vi "Template Replace.vi"() -> ()   [LabVIEW 2013]
panel:
  in  "String 6":string="fasdfas"
  out "Boolean 5":bool=TRUE
  in  "Boolean 4":bool
  out "Boolean 3":bool
  out "Numeric 2":dbl
  in  "Numeric":u16 format="%.0x"
  out "Cluster":cluster{"Boolean 2":bool}
  out "Array":string[](array[string])
  in  "Error In":errorcluster
  in  "String 5":string
  out "String 4":string
  in  "File Path Control":path
  in  "String 3":string="324"
  out "String 2":string
  in  "String":string
  out "Boolean 2":bool
  in  "Boolean":bool
  in  "Cluster 3":T1
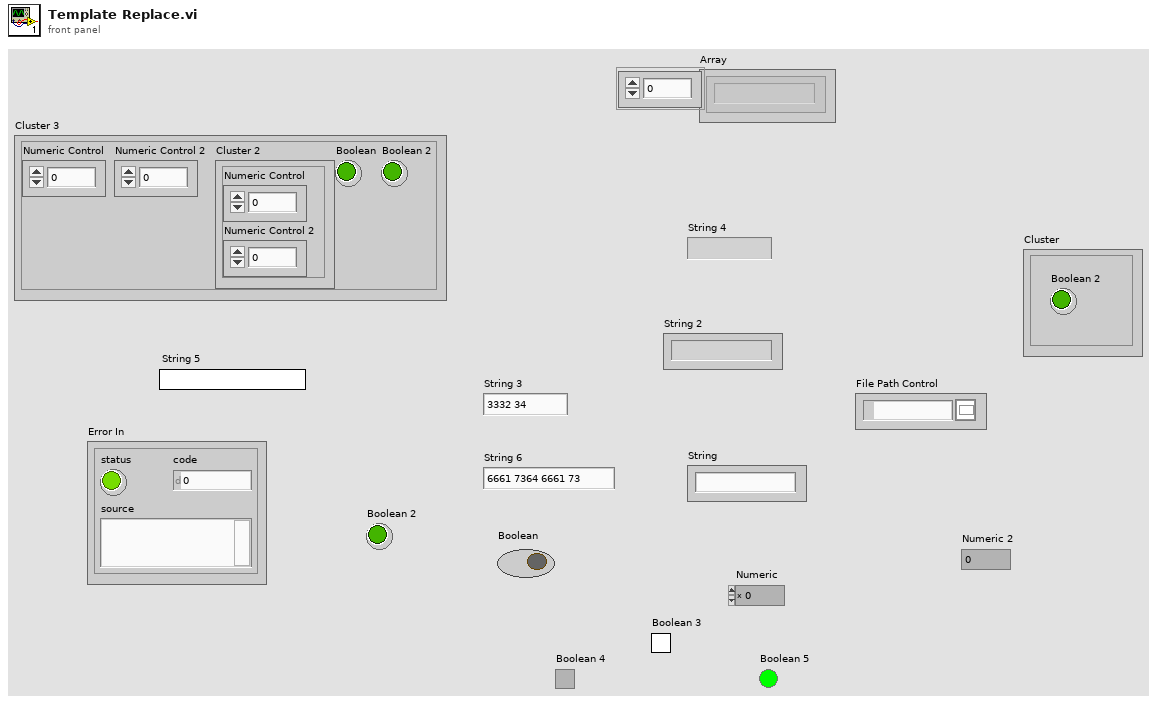
[diagram p1: front panel]
types:
  T1 = cluster{"Numeric Control":dbl, "Numeric Control 2":dbl, "Cluster 2":cluster{"Numeric Control":dbl, "Numeric Control 2":dbl}, "Boolean":bool, "Boolean 2":bool}
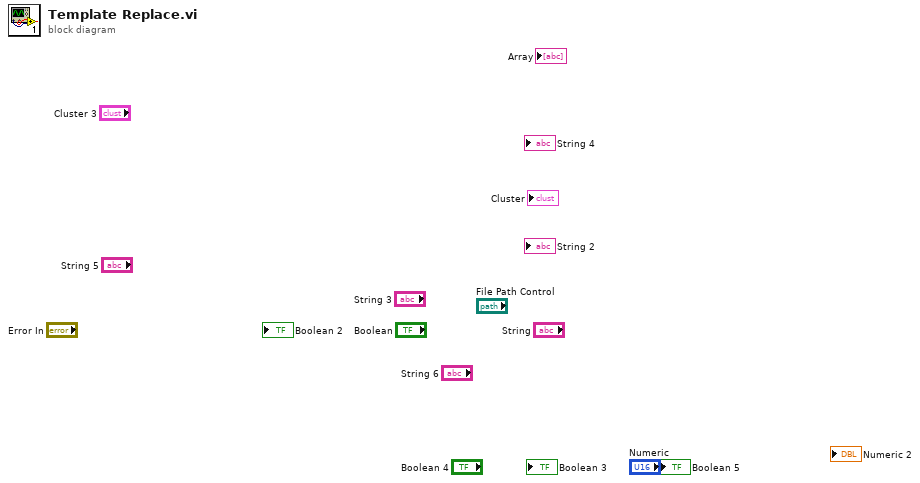
[diagram p0: block diagram]
diagram:
